vi "AI DMA Query Samples Available.vi"(0 "task in":refnum<k21>, 11 "error in":errorcluster) -> (4 "task out":refnum<k21>, 6 "samples per chan available":u32, 15 "error out":errorcluster)   [LabVIEW 2020]
doc: "Returns the number of samples per channel that are available to be read from the DMA buffer."
uses:
  <vilib>/_DAQmxBase/Internals/SSeries/Typedefs/SSeries.DMASettings.ctl
  <vilib>/_dmxb/_LVRLP/DMA.llb/DMA Read i16.vi
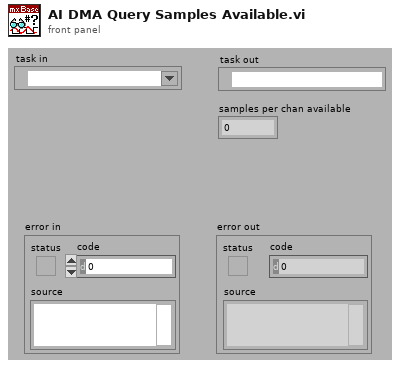
[diagram p1: front panel]
types:
  T1 = typedef "SSeries.DMASettings.ctl" = cluster{"DMA Channel":u32, "DMA Buffer in Bytes":u32, "DMA Mode":enum16{"Normal", "Ring Buffer (Continuous)", "Link Chaining", "Link Chaining (Continuous)"}, "Start DMA":bool}
  T2 = typedef "DAQmxBase Register Map Strict Type Def.ctl" = enum16{"none", "4452", "4472", "6110", "DIO32HS", "DIO96", "ESeries", "CFDAQ6004", "USB-92xx", "67xx", "SSeries", "MSeries", "USB-621x"}
  T3 = cluster{"Register Map":T2, "Acquisition Type":enum16{"none", "Analog Input", "Analog Output", "Counter Input", "Counter Output", "Digital I/O"}, "2nd Index":u32}
  T4 = typedef "DAQmxBase ESeries AI Task Type Def.ctl" = cluster{"Scan List":cluster{"Channel":u32, "Gain":enum16{"000_5", "001_0", "002_0", "005_0", "010_0", "020_0", "050_0", "100_0"}, "Polarity":enum16{"Bipolar", "Unipolar"}, "ChannelType":enum16{"Calibration", "Differential", "NRSE", "RSE", "_4", "Aux", "_6", "Ghost"}}[], "Scan Rate (Hz)":dbl, "Convert Rate (Hz)":dbl, "Number of Scans":u32, "Start Trigger":cluster{"Trigger Polarity":enum16{"Rising_Edge", "Falling_Edge"}, "Trigger Source":enum16{"Pulse", "PFI0", "PFI1", "PFI2", "PFI3", "PFI4", "PFI5", "PFI6", "PFI7", "PFI8", "PFI9", "RTSI0", "RTSI1", "RTSI2", "RTSI3", "RTSI4", "RTSI5", "RTSI6", "GPCtr0_Out", "_19", "_20", "_21", "_22", "_23", "_24", "_25", "_26", "_27", "_28", "_29", "_30", "Low"}}, "Reference Trigger":cluster{"Pretrigger Scans":u32, "Trigger Polarity":enum16{"Rising_Edge", "Falling_Edge"}, "PreTrigger Source":enum16{"Pulse", "PFI0", "PFI1", "PFI2", "PFI3", "PFI4", "PFI5", "PFI6", "PFI7", "PFI8", "PFI9", "RTSI0", "RTSI1", "RTSI2", "RTSI3", "RTSI4", "RTSI5", "RTSI6", "_18", "_19", "_20", "_21", "_22", "_23", "_24", "_25", "_26", "_27", "_28", "_29", "_30", "Low"}}, "Analog Trigger":cluster{"Analog Trig Mode":enum16{"Low Window", "High Window", "Middle Window", "_3", "High Hysteresis", "_5", "Low Hysteresis", "Disabled"}, "Analog Hi Ref":dbl, "Analog Low Ref":dbl}, "DMA":cluster{"DMA Channel":enum16{"No DMA", "Chan 1", "Chan 2", "Chan 3"}, "DMA Buffer in Bytes":u32}, "Scan Clock":cluster{"AISTARTSelect":enum16{"SI_TC", "PFI0", "PFI1", "PFI2", "PFI3", "PFI4", "PFI5", "PFI6", "PFI7", "PFI8", "PFI9", "RTSI0", "RTSI1", "RTSI2", "RTSI3", "RTSI4", "RTSI5", "RTSI6", "Pulse", "GPCtr0_Out", "_20", "_21", "_22", "_23", "_24", "_25", "_26", "_27", "_28", "_29", "_30", "Low"}, "AISTARTPolarity":enum16{"Rising_Edge", "Falling_Edge"}}, "Board Index":u32, "Timing Mode":T5, "Routes":T6[]}
  T5 = typedef "Timing Mode.ctl" = enum16{"On Demand", "Finite", "Continuous"}
  T6 = typedef "DAQmxBase export signal route typedef.ctl" = cluster{"signal (source)":enum16{"AI Sample Clock", "AI Convert Clock", "AI Start Trigger", "AI Reference Trigger", "AO Sample Clock", "AO Start Trigger", "None"}, "terminal (destination)":enum16{"PFI n", "RTSI n", "None"}, "n":i32}
  T7 = cluster{"Channel":u32, "Gain":enum16{"000_5", "001_0", "002_0", "005_0", "010_0", "020_0", "050_0", "100_0"}, "Polarity":enum16{"Bipolar", "Unipolar"}, "ChannelType":enum16{"Calibration", "Differential", "NRSE", "RSE", "_4", "Aux", "_6", "Ghost"}}[]
  T8 = typedef "MSeries.Typedef.AITask.ctl" = cluster{"Channel List":T9[], "Board Index":i32, "Number of samples":u32, "Convert Period":u32, "Sample Period":u32, "Timing Mode":T11, "Start Trigger":T12, "Sample Clock":T13, "Convert Clock":T14, "Reference Trigger":T15, "Analog Trigger":T16, "DMA Info":T17, "Routes":T6[]}
  T9 = typedef "MSeries.Typedef.AIChannelInfo.ctl" = cluster{"Channel":i32, "Range":T10, "Coupling":enum16{"DC", "AC"}, "FilterL":i32, "FilterH":i32, "Requested Range":cluster{"min":dbl, "max":dbl}, "ChannelType":enum16{"Calibration", "Differential", "NRSE", "RSE", "_4", "Aux", "_6", "Ghost"}, "Scaling":dbl[]}
  T10 = typedef "MSeries.Typedef.AIRange.ctl" = enum16{"50V to -50V", "20V to -20V", "10V to -10V", "5V to -5V", "2.5V to -2.5V", "2V to -2V", "1.25V to -1.25V", "1V to -1V", "0.5V to -0.5V", "0.25V to 0.25V", "0.2V to -0.2V", "0.1V to -0.1V"}
  T11 = typedef "MSeries.Typedef.TimingMode.ctl" = enum16{"On Demand", "Finite", "Continuous", "Hw Timed Single Point", "Invalid"}
  T12 = typedef "MSeries.Typedef.StartTrigger.ctl" = cluster{"Source":enum16{"Pulse", "PFI0", "PFI1", "PFI2", "PFI3", "PFI4", "PFI5", "PFI6", "PFI7", "PFI8", "PFI9", "RTSI0", "RTSI1", "RTSI2", "RTSI3", "RTSI4", "RTSI5", "RTSI6", "GPCtr0_Out", "GPCtr1_Out", "Star_Trigger", "PFI10", "PFI11", "PFI12", "PFI13", "PFI14", "PFI15", "RTSI7", "_28", "_29", "Analog_Trigger", "Low"}, "Polarity":enum16{"Rising_Edge", "Falling_Edge"}}
  T13 = typedef "MSeries.Typedef.ScanClock.ctl" = cluster{"Source":enum16{"SI_TC", "PFI0", "PFI1", "PFI2", "PFI3", "PFI4", "PFI5", "PFI6", "PFI7", "PFI8", "PFI9", "RTSI0", "RTSI1", "RTSI2", "RTSI3", "RTSI4", "RTSI5", "RTSI6", "Pulse", "GPCtr0_Out", "Star_Trigger", "PFI10", "PFI11", "PFI12", "PFI13", "PFI14", "PFI15", "RTSI7", "GPCtr1_Out", "SCXI_Trig1", "Analog_Trigger", "Low"}, "Polarity":enum16{"Rising_Edge", "Falling_Edge"}}
  T14 = typedef "MSeries.Typedef.ConvertClock.ctl" = cluster{"Source":enum16{"SI2TC", "PFI0", "PFI1", "PFI2", "PFI3", "PFI4", "PFI5", "PFI6", "PFI7", "PFI8", "PFI9", "RTSI0", "RTSI1", "RTSI2", "RTSI3", "RTSI4", "RTSI5", "RTSI6", "GPCtr1_Out", "GPCtr0_Out", "Star_Trigger", "PFI10", "PFI11", "PFI12", "PFI13", "PFI14", "PFI15", "RTSI7", "_28", "_29", "Analog_Trigger", "Low"}, "Polarity":enum16{"Falling_Edge", "Rising_Edge"}}
  T15 = typedef "MSeries.Typedef.ReferenceTrigger.ctl" = cluster{"Scans":u32, " Source":enum16{"Pulse", "PFI0", "PFI1", "PFI2", "PFI3", "PFI4", "PFI5", "PFI6", "PFI7", "PFI8", "PFI9", "RTSI0", "RTSI1", "RTSI2", "RTSI3", "RTSI4", "RTSI5", "RTSI6", "_18", "_19", "Star_Trigger", "PFI10", "PFI11", "PFI12", "PFI13", "PFI14", "PFI15", "RTSI7", "_28", "_29", "Analog_Trigger", "Low"}, "Polarity":enum16{"Rising_Edge", "Falling_Edge"}}
  T16 = typedef "MSeries.Typedef.AnalogTrigger.ctl" = cluster{"Mode":enum16{"Low Window", "High Window", "Middle Window", "_3", "High Hysteresis", "_5", "Low Hysteresis", "Disabled"}, "Hi Ref":dbl, "Lo Ref":dbl, "Source":enum16{"AI_Chan", "APFI0", "APFI1", "Ground"}, "Range":T10}
  T17 = typedef "MSeries.Typedef.DMAInfo.ctl" = cluster{"DMA Channel":u32, "DMA Buffer in Bytes":u32, "DMA Mode":enum16{"Normal", "Ring Buffer (Continuous)", "Link Chaining", "Link Chaining (Continuous)"}, "Transfer Size":enum16{"8 bit", "16 bit", "32 bit"}, "User":bool}
  T18 = typedef "DAQmxBase SSeries AI Task Type Def.ctl" = cluster{"Channel List":T19[], "Board Index":i32, "Task parameters":variant}
  T19 = typedef "AI Channel Info.ctl" = cluster{"Channel":i32, "Range":T20, "Coupling":enum16{"DC", "AC"}, "FilterL":i32, "FilterH":i32, "Requested Range":cluster{"min":dbl, "max":dbl}}
  T20 = typedef "AI Range.ctl" = enum16{"50V to -50V", "20V to -20V", "10V to -10V", "5V to -5V", "2.5V to -2.5V", "2V to -2V", "1.25V to -1.25V", "1V to -1V", "0.5V to -0.5V", "0.25V to 0.25V", "0.2V to -0.2V"}
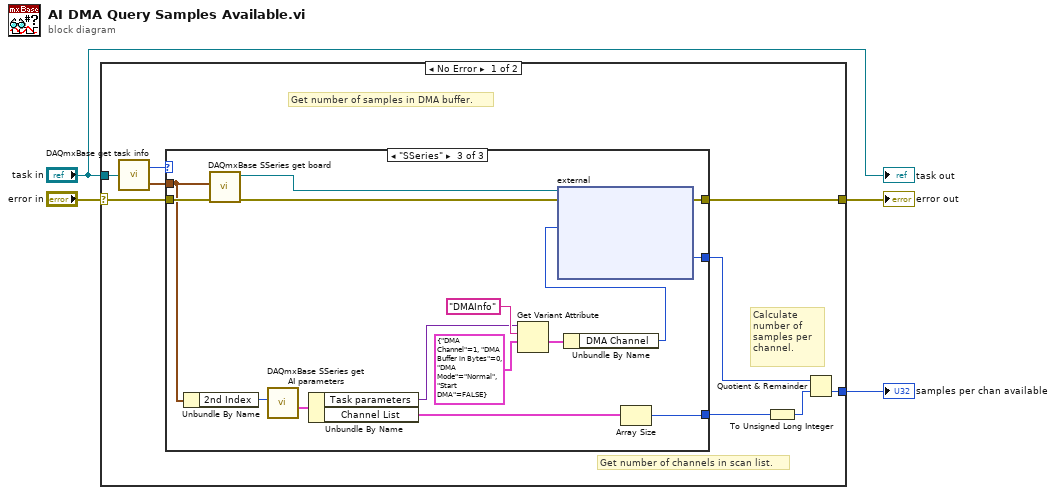
[diagram p0: block diagram]
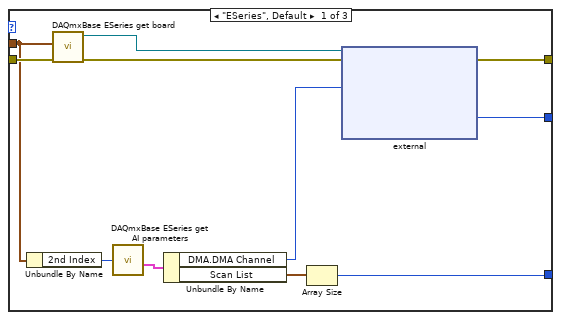
[diagram p2: hidden frame]
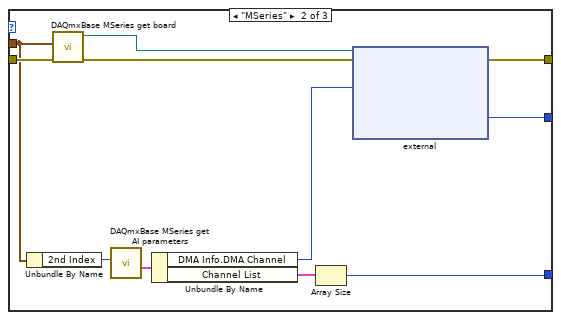
[diagram p3: hidden frame]
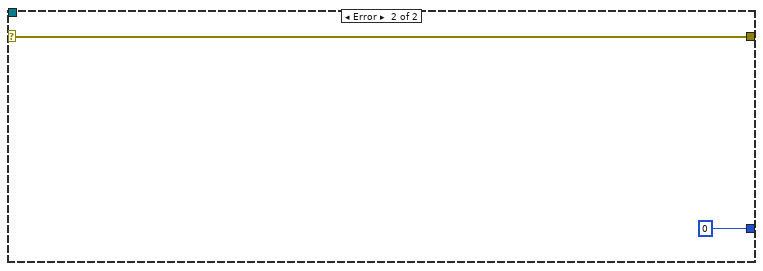
[diagram p4: hidden frame]
diagram:
  n1 = case shown="No Error" "error in" {
    selector: "error in" -> [w9 w82]
    tunnel: [w7 w82] -> w3
    tunnel: [w11 u32 0] -> w1
    tunnel: "task in" -> [w10 _]
    frame No Error {
      # "Calculate number of samples per channel."
      # "Get number of channels in scan list."
      # "Get number of samples in DMA buffer."
      n2 = call <vilib>:"DAQmxBase get task info.vi"("task/channels in"=w10) -> ("Register Map"=w6:T2, "Cluster"=w8:T3)
      n3 = case shown="\"SSeries\"" w6 {
        tunnel: [w22 w45 w70] -> w13
        tunnel: w9 -> [w21 w43 w68]
        tunnel: w8 -> [w19 w39 w61]
        tunnel: [w20 w44 w69] -> w7
        tunnel: [w14 w35 w63] -> w5
        frame "ESeries", Default {
          n4 = Unbundle By Name(w19) -> ("2nd Index"=w17:u32)
          n5 = call <vilib>:"DAQmxBase ESeries get board.vi"("error in (no error)"=w21, "Task Parameters"=w19) -> ("error out"=w24:errorcluster, "HW Exec Ref"=w23:refnum<k1>)  [unwired: 4 in]
          n6 = call <vilib>:"DAQmxBase ESeries get AI parameters.vi"("2nd Index"=w17) -> ("element"=w18:T4)  [unwired: 2 in, 1 out]
          n7 = Unbundle By Name(w18) -> ("DMA.DMA Channel"=w16:enum16{"No DMA", "Chan 1", "Chan 2", "Chan 3"}, "Scan List"=w15:T7)
          n8 = Array Size(array=w15) -> (size(s)=w14:i32)
          n9 = external ("RLP Invoke Node")(w23, w24, w16) -> (w20:errorcluster, w22:u32)  [unwired: 1 in, 2 out]
        }
        frame "MSeries" {
          n10 = Unbundle By Name(w39) -> ("2nd Index"=w38:u32)
          n11 = call <vilib>:"DAQmxBase MSeries get board.vi"("error in (no error)"=w43, "Task Parameters"=w39) -> ("error out"=w41:errorcluster, "HW Exec Ref"=w42:refnum<k1>)  [unwired: 5 in, 1 out]
          n12 = call <vilib>:"DAQmxBase MSeries get AI parameters.vi"("2nd Index"=w38) -> ("AI Task Info out"=w37:T8)  [unwired: 4 in, 2 out]
          n13 = Unbundle By Name(w37) -> ("DMA Info.DMA Channel"=w40:u32, "Channel List"=w36:T9[])
          n14 = Array Size(array=w36) -> (size(s)=w35:i32)
          n15 = external ("RLP Invoke Node")(w42, w41, w40) -> (w44:errorcluster, w45:u32)  [unwired: 1 in, 2 out]
        }
        frame "SSeries" {
          n16 = Unbundle By Name(w61) -> ("2nd Index"=w64:u32)
          n17 = call <vilib>:"DAQmxBase SSeries get board.vi"("error in (no error)"=w68, "Task Parameters"=w61) -> ("error out"=w66:errorcluster, "HW Exec Ref"=w67:refnum<k1>)  [unwired: 5 in, 1 out]
          n18 = call <vilib>:"DAQmxBase SSeries get AI parameters.vi"("2nd Index"=w64) -> ("AI Task Info out"=w65:T18)  [unwired: 4 in, 2 out]
          n19 = Unbundle By Name(w65) -> ("Task parameters"=w56:variant, "Channel List"=w62:T19[])
          n20 = Get Variant Attribute(Variant=w56, name="DMAInfo", default value (empty Variant)=T1 {"DMA Channel"=1, "DMA Buffer in Bytes"=0, "DMA Mode"=enum."Normal", "Start DMA"=FALSE} ("y")) -> (value=w60:T1)  [unwired: 1 in, 3 out]
          n21 = Unbundle By Name(w60) -> ("DMA Channel"=w57:u32)
          n22 = external ("RLP Invoke Node")(w67, w66, w57) -> (w69:errorcluster, w70:u32)  [unwired: 1 in, 2 out]
          n23 = Array Size(array=w62) -> (size(s)=w63:i32)
        }
      }
      n24 = To Unsigned Long Integer(number=w5) -> (unsigned 32bit integer=w12:u32)
      n25 = Quotient & Remainder(x=w13, y=w12) -> (floor(x/y)=w11:u32)  [unwired: 1 out]
    }
    frame Error {
    }
  }
  "error out" <- w3
  "samples per chan available" <- w1
  "task out" <- "task in"
